vi "MessungKlimadaten (SubVI).vi"(4 "Datei LV (Eingang)":refnum<file>, 6 "Datei COM (Eingang)":refnum<file>, 7 "Boolesch":bool, 8 "Fehler (Eingang, kein Fehler)":errorcluster, 9 "VISA resource name out":refnum<visa-resource-name>, 10 "Lufttemperatur [°C] (Eingang)":refnum<vi>, 11 "Luftdruck [mbar] (Eingang)":refnum<vi>) -> (0 "Fehler (Ausgang)":errorcluster, 3 "VISA-Referenz (Ausgang)":refnum<visa-resource-name>)   [LabVIEW 2014]
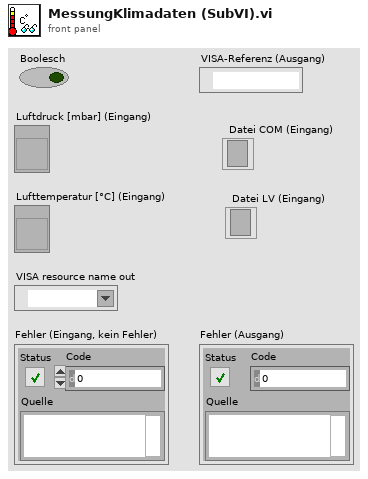
[diagram p1: front panel]
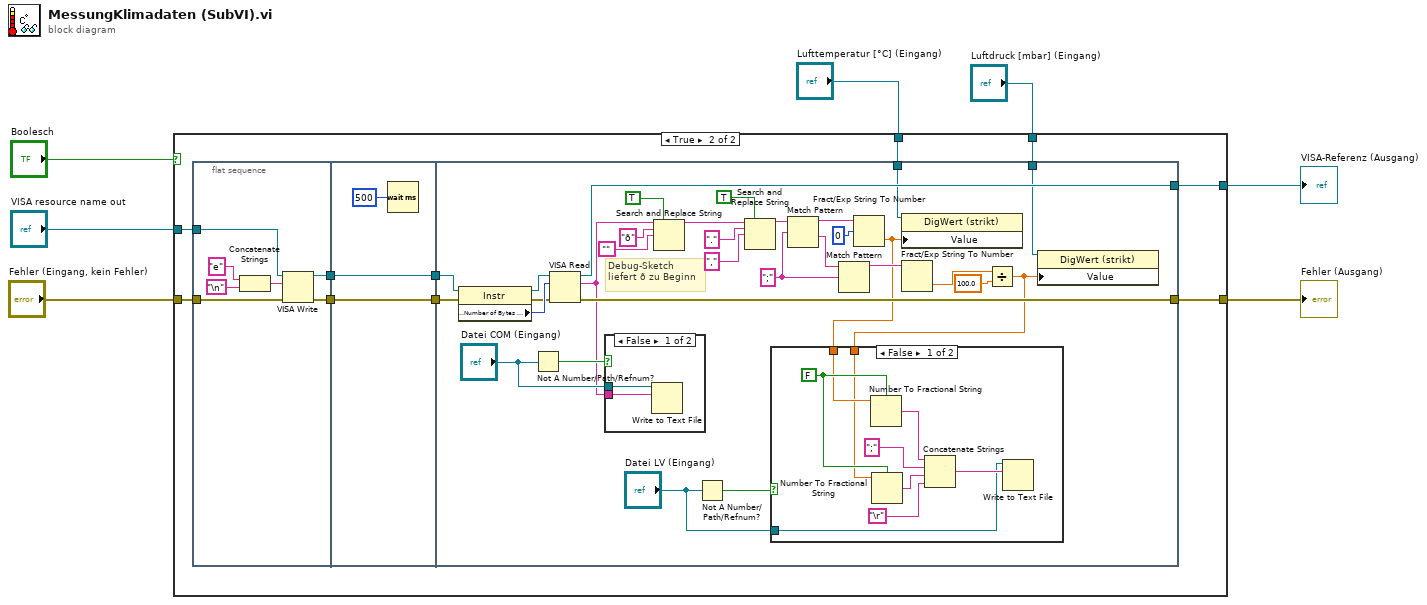
[diagram p0: block diagram]
diagram:
  n1 = case shown="True" "Boolesch" {
    tunnel: [w9 w12] -> w3
    tunnel: [w8 w13] -> w4
    tunnel: "VISA resource name out" -> [w9 w19]
    tunnel: "Fehler (Eingang, kein Fehler)" -> [w8 w18]
    tunnel: "Luftdruck [mbar] (Eingang)" -> [_ w11]
    tunnel: "Lufttemperatur [°C] (Eingang)" -> [_ w10]
    frame False {
    }
    frame True {
      n2 = flat-sequence {
        tunnel: w19 -> [w24]
        tunnel: w18 -> [w23]
        tunnel: [w26] -> w17
        tunnel: [w25] -> w16
        tunnel: w17 -> [w29]
        tunnel: w16 -> [w28]
        tunnel: [w29] -> w15
        tunnel: [w28] -> w14
        tunnel: w15 -> [w47]
        tunnel: w14 -> [w46]
        tunnel: [w49] -> w13
        tunnel: [w48] -> w12
        tunnel: w11 -> [w45]
        tunnel: w10 -> [w44]
        frame #0 {
          n3 = Concatenate Strings("e" ("String"), "\n") -> (w22:string)
          n4 = VISA Write(VISA resource name=w24, write buffer=w22, error in (no error)=w23) -> (VISA resource name out=w26:refnum<visa-resource-name>, error out=w25:errorcluster)  [unwired: 1 out]
        }
        frame #1 {
          n5 = Wait (ms)(milliseconds to wait=u32 500 ("Zu wartende ms")) -> ()  [unwired: 1 out]
        }
        frame #2 {
          w53 = ";" ("Regulärer Ausdruck")
          # "Debug-Sketch liefert ð zu Beginn"
          n6 = property class="Instr"(reference=w47, error in=w46) -> (reference out=w54:refnum<visa-resource-name>, error out=w55:errorcluster, "Serial Settings:Number of Bytes at Serial Port"=w56:u32)
          n7 = Not A Number/Path/Refnum?(number/path/refnum="Datei COM (Eingang)") -> (NaN/Path/Refnum?=w36:bool)
          n8 = VISA Read(VISA resource name=w54, byte count=w56, error in (no error)=w55) -> (VISA resource name out=w48:refnum<visa-resource-name>, read buffer=w34:string, error out=w49:errorcluster)  [unwired: 1 out]
          n9 = case shown="False" w36 {
            tunnel: "Datei COM (Eingang)" -> [w71 _]
            tunnel: w34 -> [w70 _]
            frame False {
              n10 = Write to Text File(file (use dialog)=w71, text=w70) -> ()  [unwired: 2 in, 3 out]
            }
            frame True {
            }
          }
          n11 = Search and Replace String(replace all?=TRUE ("Alle ersetzen? (F)"), input string=w34, search string="ð" ("Such-String"), replace string="") -> (result string=w38:string)  [unwired: 4 in, 3 out]
          n12 = Not A Number/Path/Refnum?(number/path/refnum="Datei LV (Eingang)") -> (NaN/Path/Refnum?=w33:bool)
          n13 = Search and Replace String(replace all?=TRUE ("Alle ersetzen? (F)"), input string=w38, search string="." ("Such-String"), replace string="," ("Ersetzungs-String (\"\")")) -> (result string=w58:string)  [unwired: 4 in, 3 out]
          n14 = Match Pattern(string=w58, regular expression=w53) -> (before substring=w41:string, after substring=w59:string)  [unwired: 1 in, 2 out]
          n15 = Match Pattern(string=w59, regular expression=w53) -> (before substring=w60:string)  [unwired: 1 in, 3 out]
          n16 = Fract/Exp String To Number(string=w41, offset=0 ("Offset")) -> (number=w32:dbl)  [unwired: 2 in, 1 out]
          n17 = property class="DigWert (strikt)"(reference=w44, "Value"=w32) -> ()  [unwired: 1 in, 2 out]
          n18 = Fract/Exp String To Number(string=w60) -> (number=w57:dbl)  [unwired: 3 in, 1 out]
          n19 = Divide(x=w57, y=100.0 ("x")) -> (x/y=w31:dbl)
          n20 = case shown="False" w33 {
            tunnel: w32 -> [w64 _]
            tunnel: w31 -> [w63 _]
            tunnel: "Datei LV (Eingang)" -> [w61 _]
            frame False {
              w66 = FALSE
              n21 = Number To Fractional String(use system decimal point (T)=w66, number=w64) -> (F-format string=w67:string)  [unwired: 2 in]
              n22 = Number To Fractional String(use system decimal point (T)=w66, number=w63) -> (F-format string=w69:string)  [unwired: 2 in]
              n23 = Concatenate Strings(w67, ";", w69, "\r") -> (w62:string)
              n24 = Write to Text File(file (use dialog)=w61, text=w62) -> ()  [unwired: 2 in, 3 out]
            }
            frame True {
            }
          }
          n25 = property class="DigWert (strikt)"(reference=w45, "Value"=w31) -> ()  [unwired: 1 in, 2 out]
        }
      }
    }
  }
  "Fehler (Ausgang)" <- w4
  "VISA-Referenz (Ausgang)" <- w3
